vi "MHX.vi"(0 "Area":dbl, 1 "MHX Tube Wall Temp":dbl, 2 "MHX Tube Diameter":dbl, 3 "Pri Cold Temp":dbl, 4 "Thermal Conductivity of FLiNaK":dbl, 5 "Pri Hot Temp":dbl, 6 "MHX Tube Wall Thickness":dbl, 8 "Pri Mass Flow":dbl, 10 "Thermal Conductivity of Hastealloy N":dbl, 11 "NDHX Tube Wall Temp":dbl, 12 "Thermal Conductivity of FLiBe":dbl, 13 "Pipe Diameter":dbl, 14 "Cp of FLiNaK":dbl, 15 "MHX Number of Tubes":dbl, 16 "FLiNaK Ave Viscosity":dbl, 17 "Sec Cold Temp":dbl, 18 "Specific Heat Capacity of FLiBe":dbl, 19 "MHX Length":dbl, 25 "Sec Hot Temp":dbl, 27 "Sec Mass Flow":dbl) -> (20 "MHX Tube Wall Temperature (K)":dbl, 21 "MHX Heat Transfer (W)":dbl)   [LabVIEW 2019]
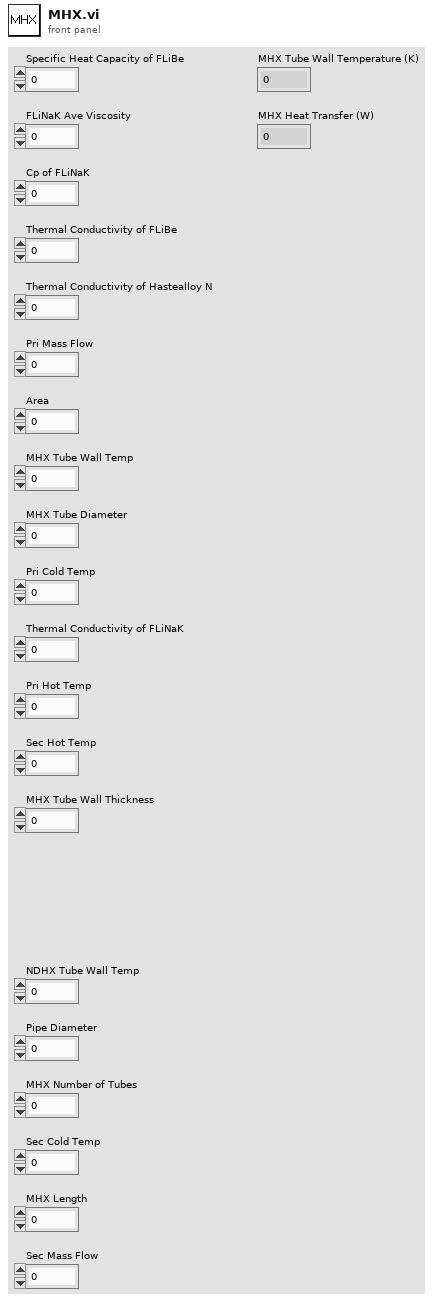
[diagram p1: front panel]
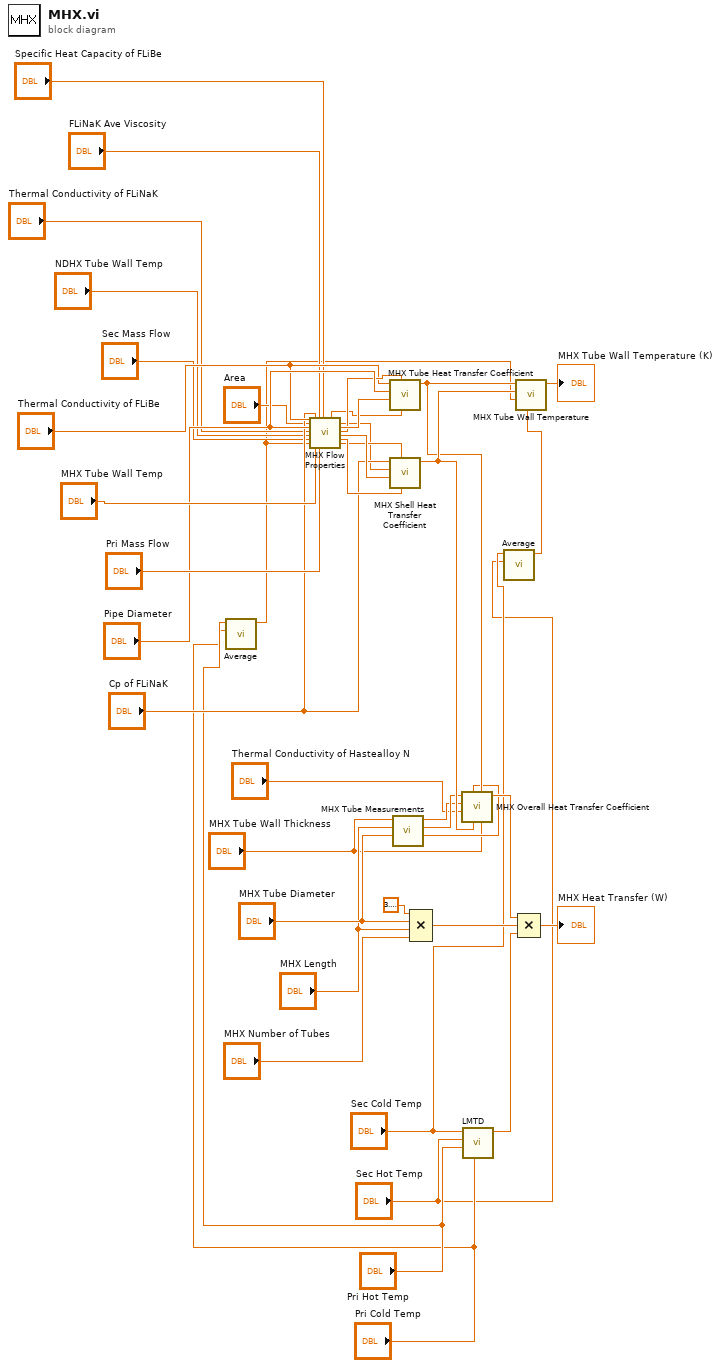
[diagram p0: block diagram]
diagram:
  n1 = call "Average.vi"("Number 2"="Pri Cold Temp", "Number 1"="Pri Hot Temp") -> ("Average"=w4:dbl)  [unwired: 9 in]
  n2 = call "MHX Flow Properties.vi"("Thermal Conductivity of FLiBe"="Thermal Conductivity of FLiBe", "Area"="Area", "Pipe Diameter"="Pipe Diameter", "Thermal Conductivity of FLiNaK"="Thermal Conductivity of FLiNaK", "NDHX Tube Wall Temp"="NDHX Tube Wall Temp", "Sec Mass Flow"="Sec Mass Flow", "Average"=w4, "Cp of FLiNaK"="Cp of FLiNaK", "MHX Tube Wall Temp"="MHX Tube Wall Temp", "FLiNaK Ave Viscosity"="FLiNaK Ave Viscosity", "Pri Mass Flow"="Pri Mass Flow", "Specific Heat Capacity of FLiBe"="Specific Heat Capacity of FLiBe") -> ("MHX Pri Re"=w19:dbl, "MHX Sec Re"=w13:dbl, "MHX Pri Phi"=w21:dbl, "MHX Pri Pr"=w20:dbl, "MHX Sec Phi"=w16:dbl, "MHX Sec Pr"=w17:dbl, "Sec Mass Flux (kg/s-m^2)"=w15:dbl)  [unwired: 7 in, 2 out]
  n3 = call "MHX Tube Heat Transfer Coefficient.vi"("MHX Pri Re"=w19, "MHX Pri Pr"=w20, "MHX Pri Phi"=w21, "Pipe Diameter"="Pipe Diameter", "Thermal Conductivity of FLiBe"="Thermal Conductivity of FLiBe") -> ("MHX Tube h"=w36:dbl)  [unwired: 6 in]
  n4 = call "MHX Shell Heat Transfer Coefficient.vi"("MHX Sec Pr"=w17, "Sec Mass Flux"=w15, "MHX Sec Phi"=w16, "MHX Sec Re"=w13, "Cp of FLiNaK"="Cp of FLiNaK") -> ("MHX Shell h"=w37:dbl)  [unwired: 6 in]
  n5 = call "MHX Tube Measurements.vi"("MHX Tube Diameter"="MHX Tube Diameter", "MHX Length"="MHX Length", "MHX Tube Wall Thickness"="MHX Tube Wall Thickness") -> ("Am (m^2)"=w24:dbl, "Ai (m^2)"=w26:dbl, "Ao (m^2)"=w25:dbl)  [unwired: 6 in]
  n6 = Compound Arithmetic op=MULTIPLY(3.141592653589793, "MHX Tube Diameter", "MHX Length", "MHX Number of Tubes") -> (w32:dbl)
  n7 = call "MHX Overall Heat Transfer Coefficient.vi"("MHX Tube Wall Thickness"="MHX Tube Wall Thickness", "MHX Tube h"=w36, "MHX Shell h"=w37, "Am"=w24, "Thermal Conductivity of Hastealloy N"="Thermal Conductivity of Hastealloy N", "Ao"=w25, "Ai"=w26) -> ("MHX Overall Heat Transfer Coefficient"=w31:dbl)  [unwired: 4 in]
  n8 = call "LMTD.vi"("Tube Cold Temp (K)"="Pri Cold Temp", "Tube Hot Temp (K)"="Pri Hot Temp", "Shell Hot Temp (K)"="Sec Hot Temp", "Shell Cold Temperature (K)"="Sec Cold Temp") -> ("LMTD (K)"=w33:dbl)  [unwired: 7 in]
  n9 = call "Average.vi"("Number 2"="Sec Hot Temp", "Number 1"="Sec Cold Temp") -> ("Average"=w1:dbl)  [unwired: 9 in]
  n10 = call "MHX Tube Wall Temperature.vi"("Sec Ave Temperature (K)"=w1, "Pri Ave Temperature (K)"=w4, "MHX Shell h"=w37, "MHX Tube h"=w36) -> ("MHX Tube Wall Temperature (K)"=→"MHX Tube Wall Temperature (K)":dbl)  [unwired: 7 in]
  n11 = Compound Arithmetic op=MULTIPLY(w31, w32, w33) -> (→"MHX Heat Transfer (W)":dbl)
